vi "CCSA RPJ SLJC PF SubVI005.vi"(11 "Datos finales":T1(array[cluster])) -> ()   [LabVIEW 2021]
uses:
  <vilib>/Utility/NIReport.llb/Report Type.ctl
  <vilib>/Utility/NIReport.llb/Append Report Text (str wrap).vi
  <vilib>/Utility/NIReport.llb/Append Image to Report (path wrap).vi
  <vilib>/Utility/NIReport.llb/NI_report.lvclass
  <vilib>/Utility/NIReport.llb/NI_ReportGenerationCore.lvlib
panel:
  out "appended path":path
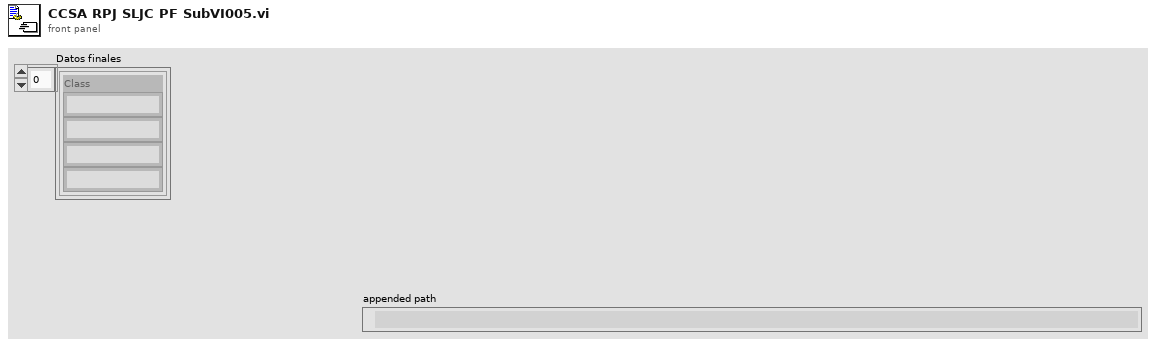
[diagram p1: front panel]
types:
  T1 = cluster{"Class":string, string, string, string}[]
  T2 = typedef "NI_ReportGenerationCore.lvlib/Report Type.ctl" = enum16{"HTML", "Word", "Excel"}
  T3 = cluster{"Charset (-1)":i16, "Weight (-1)":i16, "Name":string, "Size":string}
  T4 = cluster{"Italic":enum16{"Italic Unchanged", "Italic On", "Italic Off"}, "Strike Through":enum16{"Strike Through Unchanged", "Strike Through On", "Strike Through Off"}, "Underline":enum16{"Underline Unchanged", "Underline On", "Underline Off"}, "Bold":enum16{"Bold Unchanged", "Bold On", "Bold Off"}}
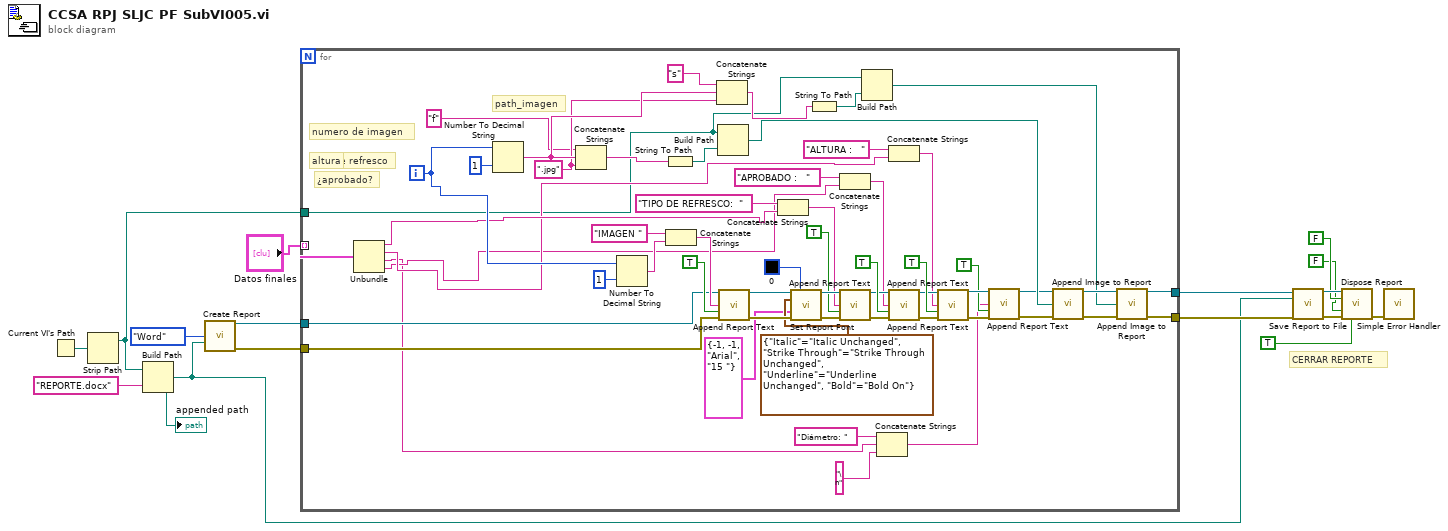
[diagram p0: block diagram]
diagram:
  # "CERRAR REPORTE"
  n1 = Current VI's Path() -> (path=w7:path)
  n2 = Strip Path(path=w7) -> (stripped path=w4:path)  [unwired: 1 out]
  n3 = Build Path(base path=w4, name or relative path="REPORTE.docx") -> (appended path=w8:path)
  "appended path" <- w8
  n4 = call <vilib>:"Create Report.vi"("report type"=Report_Type."Word", "template (empty)"=w8) -> ("report out"=w3:refnum<class "NI_report.lvclass">, "error out"=w2:errorcluster)  [unwired: 12 in]
  n5 = for {
    tunnel: "Datos finales" -> [w73] mode=indexing
    tunnel: [w36] -> w11
    tunnel: [w35] -> w10
    tunnel: w4 -> [w29]
    tunnel: w3 -> [w40]
    tunnel: w2 -> [w39]
    i -> [w72]
    w32 = ".jpg" ("string")
    # "path_imagen"
    # "altura"
    # "¿aprobado?"
    # "tipo de refresco"
    # "numero de imagen"
    n6 = Unbundle(w73) -> ("Class"=w71:string, w70:string, w20:string, w21:string)
    n7 = Number To Decimal String(number=w72, width (-)=i16 1) -> (decimal integer string=w33:string)
    n8 = Concatenate Strings("f" ("string"), w33, w32) -> (w43:string)
    n9 = Number To Decimal String(number=w72, width (-)=i16 1) -> (decimal integer string=w61:string)
    n10 = String To Path(string=w43) -> (path=w44:path)
    n11 = Concatenate Strings("IMAGEN " ("text"), w61) -> (w60:string)
    n12 = Concatenate Strings("s" ("string"), w33, w32) -> (w30:string)
    n13 = Build Path(base path=w29, name or relative path=w44) -> (appended path=w41:path)
    n14 = call-poly <vilib>:"Append Report Text.vi"("report in"=w40, "text"=w60, "append on new line? (F)"=TRUE, "error in (no error)"=w39) -> ("report out"=w68:refnum<class "NI_report.lvclass">, "error out"=w67:errorcluster)  [unwired: 8 in, 2 out]
    n15 = Concatenate Strings("TIPO DE REFRESCO:  " ("text"), w71) -> (w55:string)
    n16 = call-dynamic "Set Report Font.vi"("report in"=w68, "text color (unchanged)"=u32 0, "text options"=T4 {"Italic"=enum."Italic Unchanged", "Strike Through"=enum."Strike Through Unchanged", "Underline"=enum."Underline Unchanged", "Bold"=enum."Bold On"}, "font settings"=T3 {"Charset (-1)"=-1, "Weight (-1)"=-1, "Name"="Arial", "Size"="15 "}, "error in (no error)"=w67) -> ("report out"=w59:refnum<class "NI_report.lvclass">, "error out"=w58:errorcluster)  [unwired: 8 in, 1 out]
    n17 = String To Path(string=w30) -> (path=w31:path)
    n18 = Concatenate Strings("APROBADO :   " ("text"), w21) -> (w46:string)
    n19 = call-poly <vilib>:"Append Report Text.vi"("report in"=w59, "text"=w55, "append on new line? (F)"=TRUE, "error in (no error)"=w58) -> ("report out"=w50:refnum<class "NI_report.lvclass">, "error out"=w47:errorcluster)  [unwired: 8 in, 2 out]
    n20 = Build Path(base path=w29, name or relative path=w31) -> (appended path=w28:path)
    n21 = Concatenate Strings("Diámetro: " ("text"), w20, "\n" ("text")) -> (w19:string)
    n22 = Concatenate Strings("ALTURA :   " ("text"), w70) -> (w45:string)
    n23 = call-poly <vilib>:"Append Report Text.vi"("report in"=w50, "text"=w46, "append on new line? (F)"=TRUE, "error in (no error)"=w47) -> ("report out"=w49:refnum<class "NI_report.lvclass">, "error out"=w48:errorcluster)  [unwired: 8 in, 2 out]
    n24 = call-poly <vilib>:"Append Report Text.vi"("report in"=w49, "text"=w45, "append on new line? (F)"=TRUE, "error in (no error)"=w48) -> ("report out"=w24:refnum<class "NI_report.lvclass">, "error out"=w27:errorcluster)  [unwired: 8 in, 2 out]
    n25 = call-poly <vilib>:"Append Report Text.vi"("report in"=w24, "text"=w19, "append on new line? (F)"=TRUE, "error in (no error)"=w27) -> ("report out"=w25:refnum<class "NI_report.lvclass">, "error out"=w26:errorcluster)  [unwired: 8 in, 2 out]
    n26 = call-poly <vilib>:"Append Image to Report.vi"("report in"=w25, "path or URL of image"=w41, "error in (no error)"=w26) -> ("report out"=w38:refnum<class "NI_report.lvclass">, "error out"=w37:errorcluster)  [unwired: 9 in, 2 out]
    n27 = call-poly <vilib>:"Append Image to Report.vi"("report in"=w38, "path or URL of image"=w28, "error in (no error)"=w37) -> ("report out"=w36:refnum<class "NI_report.lvclass">, "error out"=w35:errorcluster)  [unwired: 9 in, 2 out]
  }
  n28 = call-dynamic "Save Report to File.vi"("report in"=w11, "report file path"=w8, "error in (no error)"=w10) -> ("report out"=w14:refnum<class "NI_report.lvclass">, "error out"=w15:errorcluster)  [unwired: 11 in]
  n29 = call-dynamic "Dispose Report.vi"("report in"=w14, "wait until printing completed? (T)"=FALSE, "save changes? (F)"=FALSE, "error in (no error)"=w15, "close report? (T)"=TRUE) -> ("error out"=w16:errorcluster)  [unwired: 10 in]
  n30 = call <vilib>:"Simple Error Handler.vi"("error in (no error)"=w16) -> ()  [unwired: 4 in, 5 out]
